vi "Drive to Location.vi"(8 "power in":dbl, 10 "y":dbl, 11 "x":dbl) -> (0 "power out":dbl)   [LabVIEW 2017]
uses:
  <vilib>/Rock Robotics/WPI/RobotDrive/WPI_RobotDriveArcadeDrive_Standard(NoSaturation).vi
  Robot Global Data.vi
panel:
  out "distance left":dbl
  out "x off":dbl
  out "y off":dbl
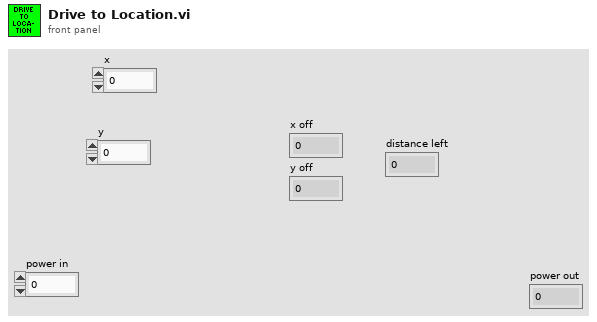
[diagram p1: front panel]
types:
  T1 = cluster{"Yaw":dbl, "Roll":dbl, "Pitch":dbl, "Heading":dbl, "Fused Heading":dbl}
  T2 = typedef "WPI_RobotDriveDevRef.ctl" = cluster{"DevStatus":errorcluster, "Motors[]":T3[], "Square Inputs":bool, "Max Output":dbl}
  T3 = typedef "WPI_MotorControlDeviceRef.ctl" = cluster{"DeviceStatus":errorcluster, "Type":T4, "PWM":cluster{"PWM Channel":T5, "DeadBand":T6}, "CAN":cluster{"Device Number":u8, "SetOutput VI Ref":variant, "GetOutput VI Ref":variant, "Enable VI Ref":variant, "Disable VI Ref":variant, "Data":variant}, "Invert":bool, "DIO PWM":cluster{"PWM \"Enable\" Channel":T5, "DIOChannel":T7, "PWM Rate":dbl}}
  T4 = typedef "WPI_MotorControlType.ctl" = enum16{"PWM", "CAN", "DIO PWM"}
  T5 = typedef "FPGA_DIOPWMChannel.ctl" = enum8{"PWM 0", "PWM 1", "PWM 2", "PWM 3", "PWM 4", "PWM 5", "PWM 6", "PWM 7", "PWM 8", "PWM 9", "PWM MXP 0", "PWM MXP 1", "PWM MXP 2", "PWM MXP 3", "PWM MXP 4", "PWM MXP 5", "PWM MXP 6", "PWM MXP 7", "PWM MXP 8", "PWM MXP 9", "Invalid"}
  T6 = typedef "WPI_PWMDeadband.ctl" = cluster{"Name":string, "maxPositivePwm":i32, "minPositivePwm":i32, "centerPwm":i32, "maxNegativePwm":i32, "minNegativePwm":i32, "angularRange":u16}
  T7 = typedef "FPGA_DIOChannel.ctl" = enum8{"DIO 0", "DIO 1", "DIO 2", "DIO 3", "DIO 4", "DIO 5", "DIO 6", "DIO 7", "DIO 8", "DIO 9", "DIO MXP 0", "DIO MXP 1", "DIO MXP 2", "DIO MXP 3", "DIO MXP 4", "DIO MXP 5", "DIO MXP 6", "DIO MXP 7", "DIO MXP 8", "DIO MXP 9", "DIO MXP 10", "DIO MXP 11", "DIO MXP 12", "DIO MXP 13", "DIO MXP 14", "DIO MXP 15", "SPI Port CS1", "SPI Port CS2", "SPI Port CS3", "SPI Port MISO", "SPI Port MOSI", "Invalid"}
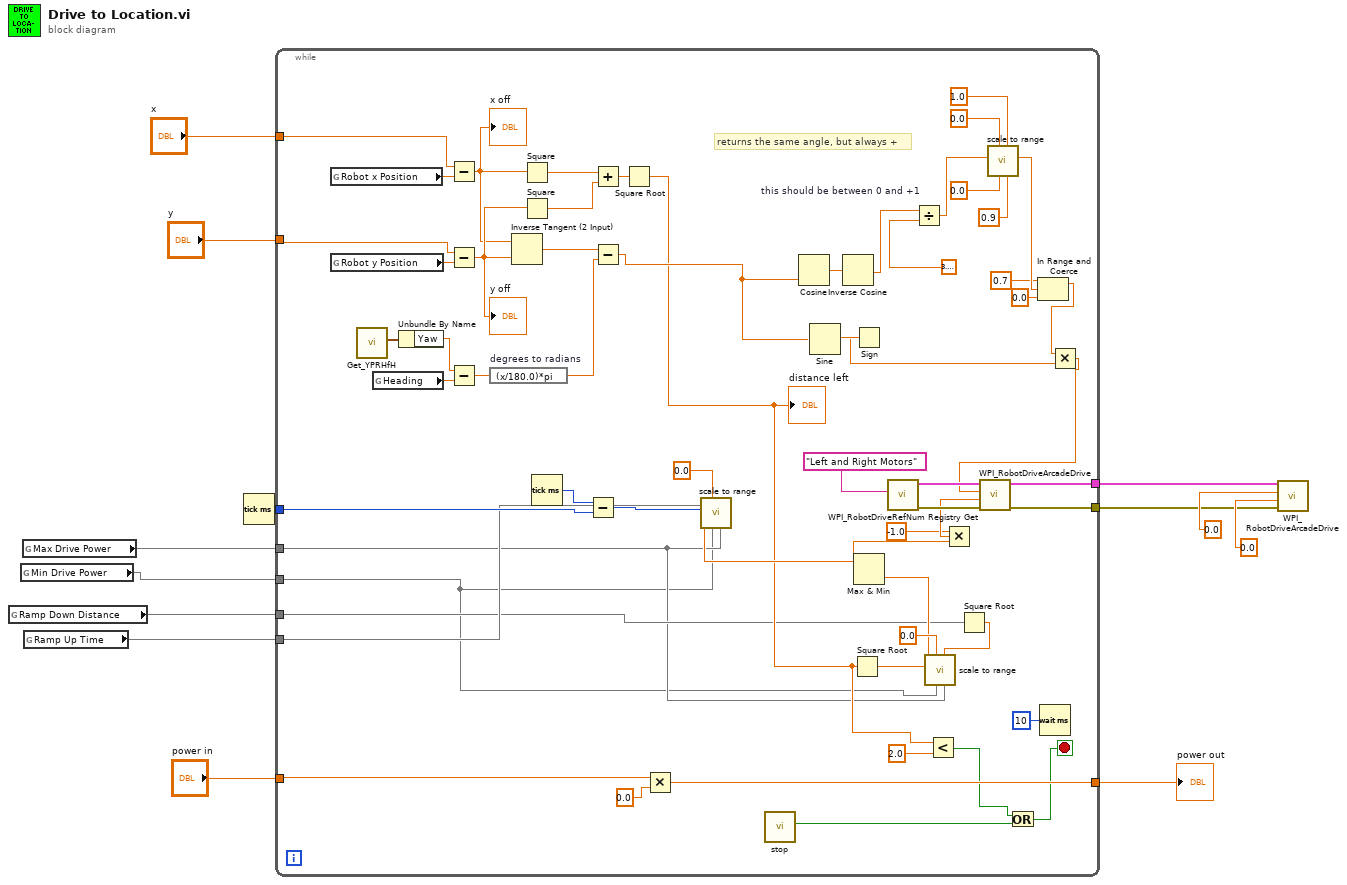
[diagram p0: block diagram]
diagram:
  n1 = global read "Robot Global Data.vi" "Ramp Down Distance"() -> (w3)
  n2 = global read "Robot Global Data.vi" "Min Drive Power"() -> (w1)
  n3 = global read "Robot Global Data.vi" "Max Drive Power"() -> (w2)
  n4 = global read "Robot Global Data.vi" "Ramp Up Time"() -> (w4)
  n5 = Tick Count (ms)() -> (millisecond timer value=w9:u32)
  n6 = while {
    tunnel: [w71] -> w11
    tunnel: [w70] -> w10
    tunnel: w9 -> [w64]
    tunnel: [w24] -> w5
    tunnel: "power in" -> [w57]
    tunnel: "y" -> [w36]
    tunnel: "x" -> [w35]
    tunnel: w4 -> [w22]
    tunnel: w3 -> [w20]
    tunnel: w2 -> [w19]
    tunnel: w1 -> [w18]
    stop <- w14 stop-if-true
    # "returns the same angle, but always +"
    n7 = global read "Robot Global Data.vi" "Robot x Position"() -> (w30:dbl)
    n8 = global read "Robot Global Data.vi" "Robot y Position"() -> (w29:dbl)
    n9 = call <vilib>:"Get_YPRHfH.vi"() -> ("YRPHfH"=w56:T1)  [unwired: 11 in]
    n10 = global read "Robot Global Data.vi" "Heading"() -> (w52:dbl)
    n11 = Unbundle By Name(w56) -> ("Yaw"=w53:dbl)
    n12 = Subtract(x=w35, y=w30) -> (x-y=w33:dbl)
    "x off" <- w33
    n13 = Subtract(x=w36, y=w29) -> (x-y=w34:dbl)
    "y off" <- w34
    n14 = Subtract(x=w53, y=w52) -> (x-y=w39:dbl)
    n15 = expression code="(x/180.0)*pi" "degrees to radians"(w39) -> (w40:dbl)
    n16 = Inverse Tangent (2 Input)(1:w34, 2:w33) -> (0:w38:dbl)
    n17 = Square(x=w33) -> (x^2=w43:dbl)
    n18 = Square(x=w34) -> (x^2=w44:dbl)
    n19 = Tick Count (ms)() -> (millisecond timer value=w63:u32)
    n20 = Subtract(x=w63, y=w64) -> (x-y=w58:u32)
    n21 = Add(x=w43, y=w44) -> (x+y=w42:dbl)
    n22 = Subtract(x=w38, y=w40) -> (x-y=w41:dbl)
    n23 = Square Root(x=w42) -> (sqrt(x)=w32:dbl)
    "distance left" <- w32
    n24 = Multiply(x=w57, y=0.0) -> (x*y=w24:dbl)
    n25 = call "scale to range.vi"("Max"=w19, "High"=w22, "Min"=w18, "Low"=0.0, "In Signal"=w58) -> ("Output signal"=w60:dbl)  [unwired: 6 in]
    n26 = call "stop.vi"() -> ("Boolean"=w16:bool)  [unwired: 11 in]
    n27 = Cosine(x=w41) -> (cos(x)=w55:dbl)
    n28 = Sine(x=w41) -> (sin(x)=w54:dbl)
    n29 = Inverse Cosine(1:w55) -> (0:w50:dbl)
    n30 = Square Root(x=w32) -> (sqrt(x)=w66:dbl)
    n31 = Sign(1:w54) -> (0:w45:dbl)
    n32 = call <vilib>:"WPI_RobotDriveRefNum Registry Get.vi"("refnum name"="Left and Right Motors") -> ("error out"=w73:errorcluster, "RobotDriveDevRef"=w72:T2)  [unwired: 1 in, 8 out]
    n33 = Divide "this should be between 0 and +1"(x=w50, y=3.141592653589793) -> (x/y=w49:dbl)
    n34 = Less?(x=w32, y=2.0) -> (x < y?=w15:bool)
    n35 = Square Root(x=w20) -> (sqrt(x)=w21:dbl)
    n36 = call "scale to range.vi"("Max"=w19, "High"=w21, "Min"=w18, "Low"=0.0, "In Signal"=w66) -> ("Output signal"=w61:dbl)  [unwired: 6 in]
    n37 = Max & Min(x=w60, y=w61) -> (min(x,y)=w59:dbl)  [unwired: 1 out]
    n38 = Multiply(x=-1.0, y=w59) -> (x*y=w69:dbl)
    n39 = call "scale to range.vi"("Max"=0.9, "High"=1.0, "Min"=0.0, "Low"=0.0, "In Signal"=w49) -> ("Output signal"=w28:dbl)  [unwired: 6 in]
    n40 = Or(x=w15, y=w16) -> (x .or. y?=w14:bool)
    n41 = In Range and Coerce(upper limit=0.7, x=w28, lower limit=0.0) -> (coerced(x)=w27:dbl)  [unwired: 1 out]
    n42 = Wait (ms)(milliseconds to wait=u32 10) -> ()  [unwired: 1 out]
    n43 = Multiply(x=w27, y=w45) -> (x*y=w37:dbl)
    n44 = call-poly <vilib>:"WPI_RobotDriveArcadeDrive.vi"("error in (no error)"=w73, "Y axis value"=w69, "X axis value"=w37, "RobotDriveDevRef"=w72) -> ("error out"=w71:errorcluster, "RobotDriveDevRef"=w70:T2)  [unwired: 6 out]
  }
  "power out" <- w5
  n45 = call-poly <vilib>:"WPI_RobotDriveArcadeDrive.vi"("error in (no error)"=w11, "Y axis value"=0.0 ("X axis value"), "X axis value"=0.0, "RobotDriveDevRef"=w10) -> ()  [unwired: 8 out]
